vi "Calibration.vi"(8 "error in (no error)":errorcluster) -> (0 "error out":errorcluster, 2 "Cal Success":bool)   [LabVIEW 2018]
uses:
  Microfontest/Peiker_Stepped Sweep Settings.ctl
  <vilib>/addons/_NISVFA/_Shared subVIs/Controls/svc_DSA Channel Settings.ctl
  <vilib>/addons/_NISVFA/_Shared subVIs/Controls/svc_Channel Info.ctl
  <vilib>/addons/_NISVFA/_Shared subVIs/Controls/svc_Engineering Units Text Ring.ctl
  <vilib>/addons/_NISVFA/_Shared subVIs/Controls/svc_Weighting Filter Text Ring.ctl
panel:
  out "FrequencyList Output Level":T1(graph)
  in  "Cancel":bool
  out "calibrated sensor sensitivity [mV/Pa] 2":dbl
  in  "Ret":bool
  in  "Cal":bool
  out "Fundamental Amplitude":T2(graph) caption="Fundamental-Amplitude"
  in  "Freq List file":path=path "D:/Valeo/Micriphone Test/Config/ME79_FreqList_New.csv"
  out "correctedFreqList":T1(array[cluster])
  in  "CalSettings":T3={"SollPegel[dBSPL]"=114, "maxDeviationRef[dB]"=2.0, "maxDeviation[dB]"=2.0, "maxRuns"=20, "RefFrequency[Hz]"=94, "Wait[ms]"=0} {"maxDeviation[dB]" format="%.2f"; "maxDeviationRef[dB]" format="%.2f"}
  out "calibrated sensor sensitivity [mV/Pa]":dbl=nan format="%.2g"
  out "power spectrum":cluster{"x0":dbl, "dx":dbl, "magnitude":dbl[]}(graph)
  in  "calibration settings":T4={"calibration value [dB SPL]"=94.0, "calibration frequency [Hz]"=1000.0}
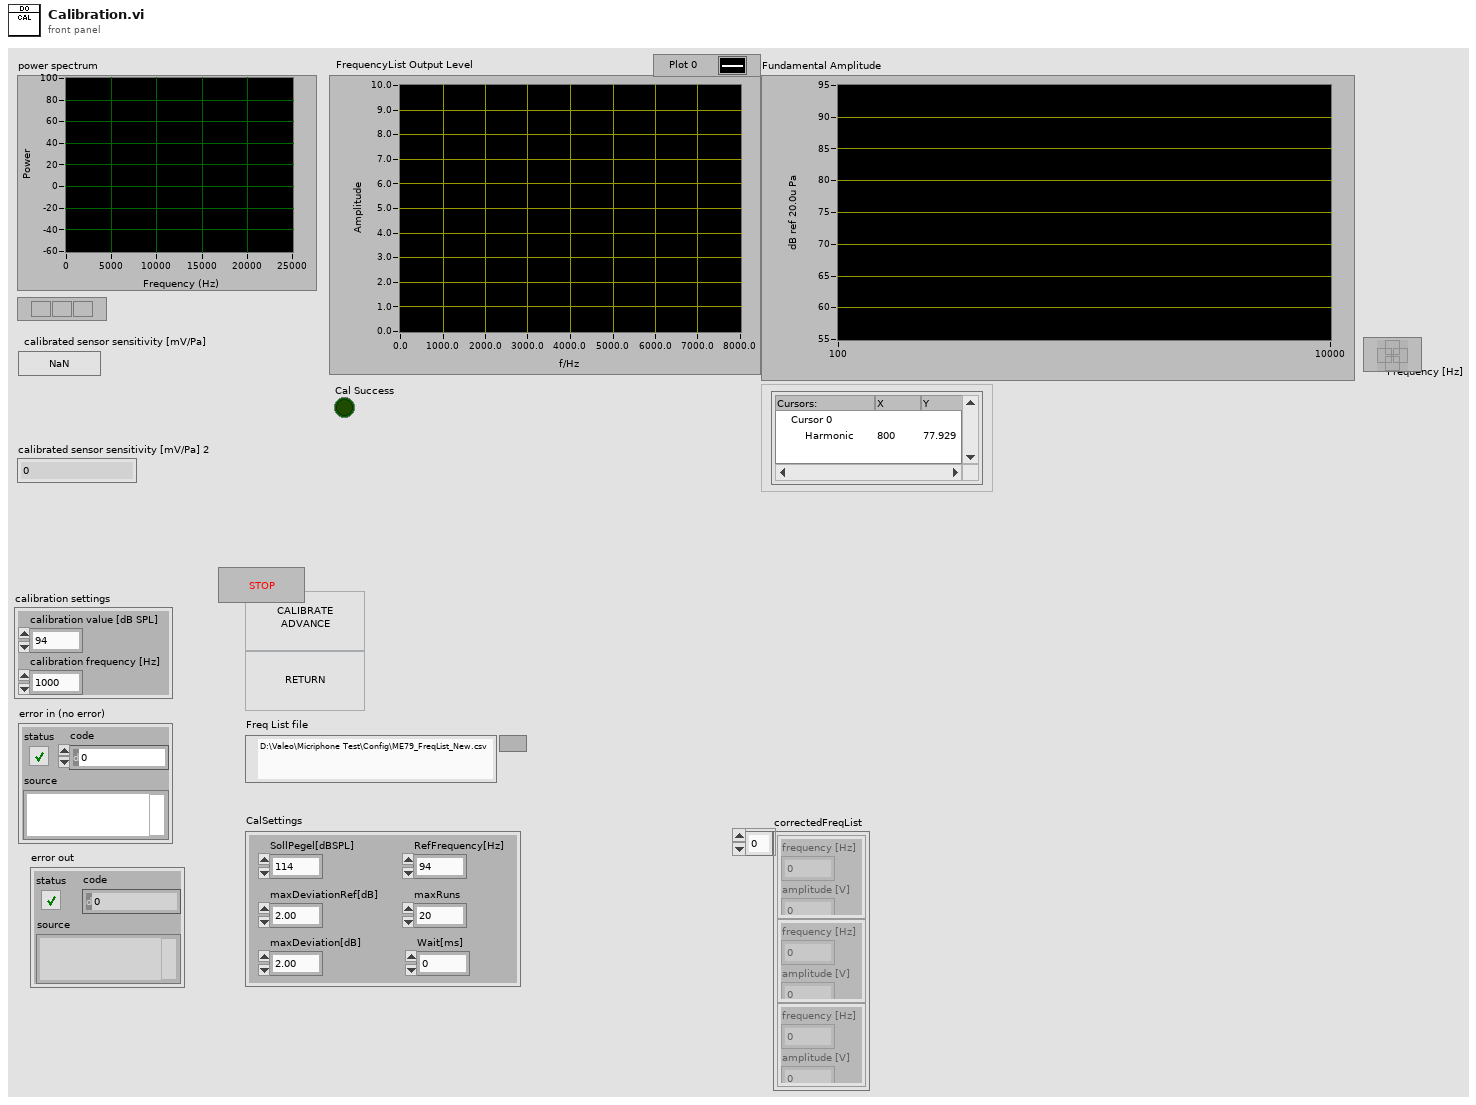
[diagram p1: front panel]
types:
  T1 = cluster{"frequency [Hz]":dbl, "amplitude [V]":dbl}[]
  T2 = cluster{"frequency [Hz]":dbl[], "amplitude":dbl[]}
  T3 = cluster{"SollPegel[dBSPL]":i32, "maxDeviationRef[dB]":dbl, "maxDeviation[dB]":dbl, "maxRuns":i32, "RefFrequency[Hz]":i32, "Wait[ms]":i32}
  T4 = cluster{"calibration value [dB SPL]":dbl, "calibration frequency [Hz]":dbl}
  T5 = typedef "Peiker_Stepped Sweep Settings.ctl" = cluster{"Input Settings":cluster{"IEPE min time to settle [s]":dbl, "Responce Channel Settings":cluster{"DSA response channel settings":T6, "response channel info":T7, "AI response settings":cluster{"response channel":tag, "max value [V]":dbl, "min value [V]":dbl, "terminal configuration":i32}}, "Stimulus Channel Settings":cluster{"AI stimulus settings":cluster{"stimulus channel":tag, "max value [V]":dbl, "min value [V]":dbl, "terminal configuration":i32}, "DSA stimulus channel settings":T6, "stimulus channel info":T7}}, "Output Settings":cluster{"AO source settings":cluster{"excitation channel":tag, "max value [V]":dbl, "min value [V]":dbl, "terminal configuration":i32}}}
  T6 = typedef "svc_DSA Channel Settings.ctl" = cluster{"coupling":i32, "enable IEPE excitation":bool, "IEPE current [mA]":dbl}
  T7 = typedef "svc_Channel Info.ctl" = cluster{"sensor sensitivity":dbl, "engineering units":T8, "dB reference":dbl, "custom label":string, "weighting filter":T9, "pregain":dbl}
  T8 = typedef "svc_Engineering Units Text Ring.ctl" = u16
  T9 = typedef "svc_Weighting Filter Text Ring.ctl" = u16
  T10 = enum16{"Left Button", "Center Button", "Right Button", "Window Close"}
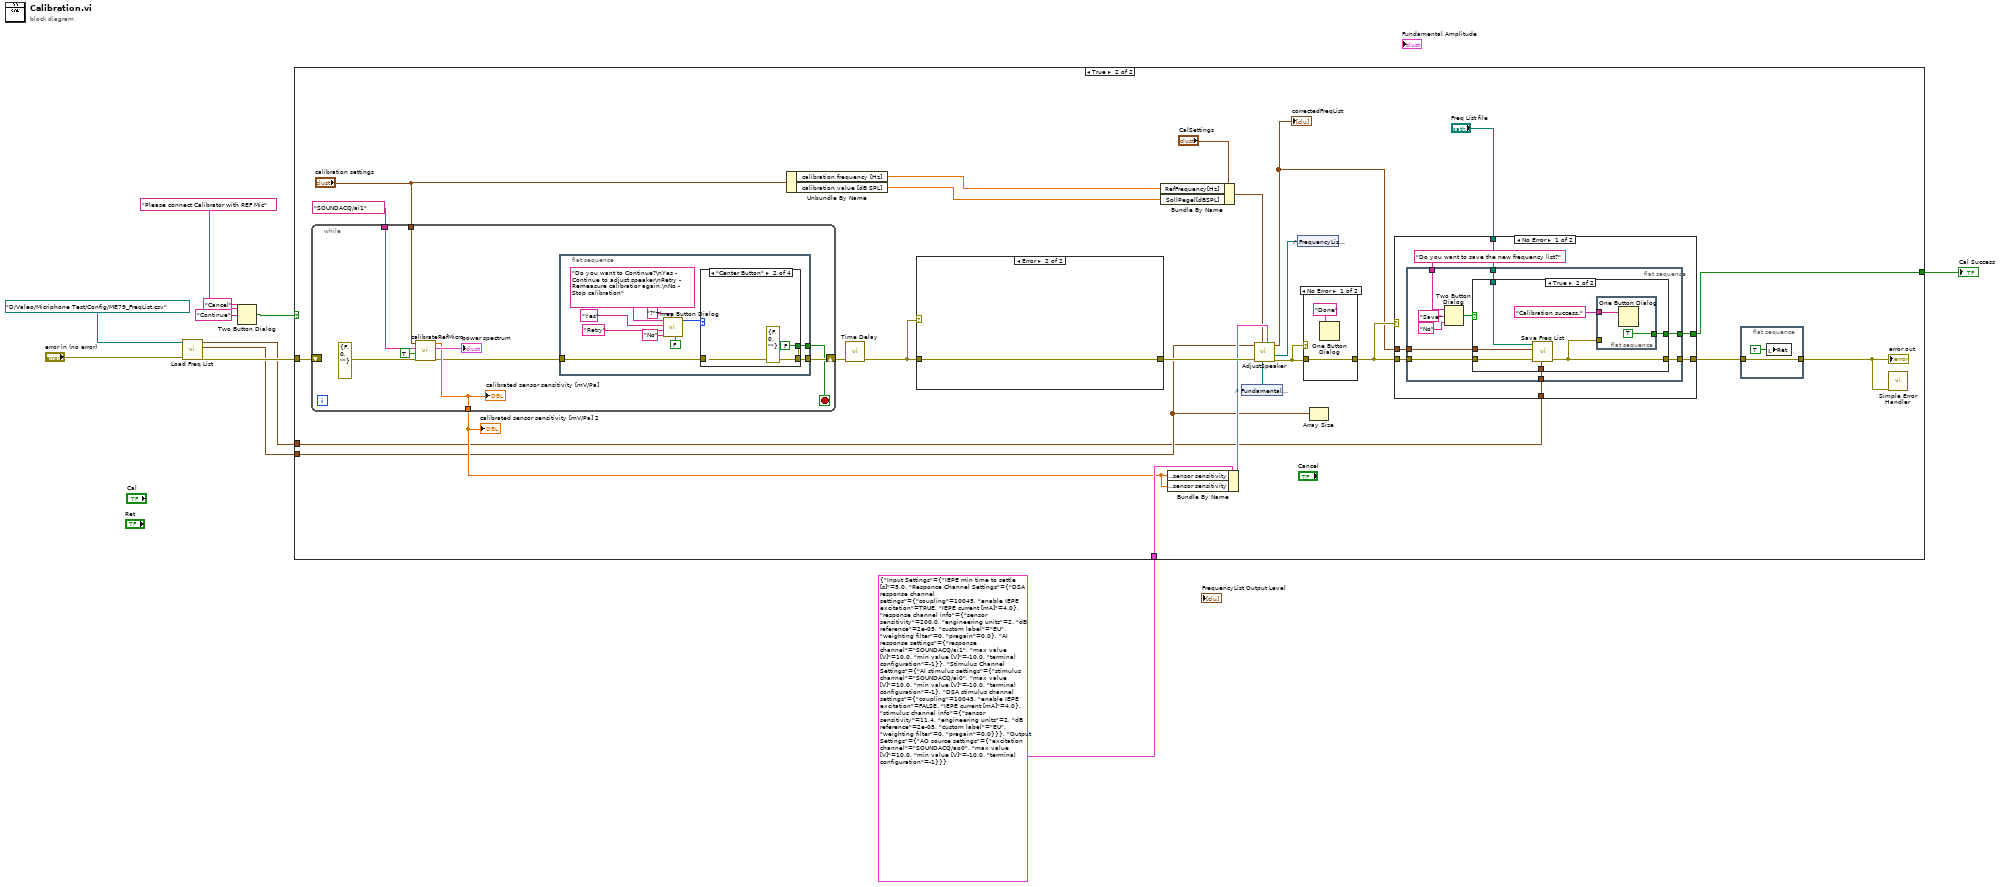
[diagram p0: block diagram]
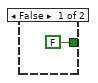
[diagram p2: hidden frame]
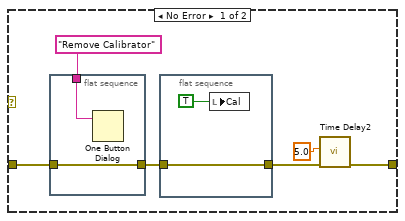
[diagram p3: hidden frame]
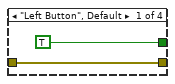
[diagram p4: hidden frame]
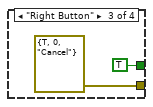
[diagram p5: hidden frame]
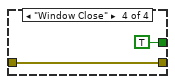
[diagram p6: hidden frame]
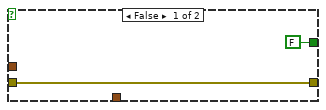
[diagram p7: hidden frame]
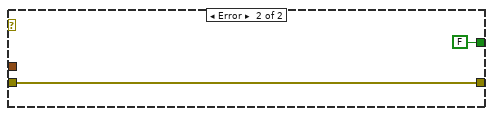
[diagram p8: hidden frame]
diagram:
  n1 = call "Load Freq List.vi"("error in (no error)"="error in (no error)", "Freq List file"=path "D:/Valeo/Micriphone Test/Config/ME79_FreqList.csv" ("dup path")) -> ("error out"=w7:errorcluster, "Frequency List"=w6:T1, "Spec List"=w1:cluster{"Lower":dbl, "Upper":dbl}[])  [unwired: 5 in, 2 out]
  n2 = Two Button Dialog(message="Please connect Calibrator with REF Mic", 1:"Cancel" ("F button name (\"Cancel\")"), 2:"Continue" ("T button name (\"OK\")")) -> (T button?=w10:bool)
  n3 = case shown="True" w10 {
    tunnel: w7 -> [_ w31]
    tunnel: w6 -> [_ w15]
    tunnel: T5 {"Input Settings"={"IEPE min time to settle [s]"=5.0, "Responce Channel Settings"={"DSA response channel settings"={"coupling"=10045, "enable IEPE excitation"=TRUE, "IEPE current [mA]"=4.0}, "response channel info"={"sensor sensitivity"=200.0, "engineering units"=2, "dB reference"=2e-05, "custom label"="EU", "weighting filter"=0, "pregain"=0.0}, "AI response settings"={"response channel"="SOUNDACQ/ai1", "max value [V]"=10.0, "min value [V]"=-10.0, "terminal configuration"=-1}}, "Stimulus Channel Settings"={"AI stimulus settings"={"stimulus channel"="SOUNDACQ/ai0", "max value [V]"=10.0, "min value [V]"=-10.0, "terminal configuration"=-1}, "DSA stimulus channel settings"={"coupling"=10045, "enable IEPE excitation"=FALSE, "IEPE current [mA]"=4.0}, "stimulus channel info"={"sensor sensitivity"=11.4, "engineering units"=2, "dB reference"=2e-05, "custom label"="EU", "weighting filter"=0, "pregain"=0.0}}}, "Output Settings"={"AO source settings"={"excitation channel"="SOUNDACQ/ao0", "max value [V]"=10.0, "min value [V]"=-10.0, "terminal configuration"=-1}}} ("Peiker_Stepped Sweep Settings") -> [_ w33]
    tunnel: [FALSE w17] -> w4
    tunnel: w1 -> [_ w14]
    frame False {
    }
    frame True {
      n4 = while {
        tunnel: tag "SOUNDACQ/ai1" ("DAQmx physical channel") -> [w56]
        tunnel: [w53] -> w30
        tunnel: "calibration settings" -> [w52]
        shift-right: [w49] -> w35
        shift-left: w31 -> [_]
        stop <- w50 stop-if-true
        n5 = call "calibrateRefMicro.vi"("error in (no error)"=errorcluster {"status"=FALSE, "code"=0, "source"=""} ("error out"), "enable IEPE excitation (F)"=TRUE, "DAQmx physical channel"=w56, "calibration settings"=w52) -> ("error out"=w51:errorcluster, "power spectrum"=→"power spectrum":cluster{"x0":dbl, "dx":dbl, "magnitude":dbl[]}, "calibrated sensor sensitivity [mV/Pa]"=w53:dbl)  [unwired: 5 in]
        "calibrated sensor sensitivity [mV/Pa]" <- w53
        n6 = flat-sequence {
          tunnel: w51 -> [w58]
          tunnel: [w59] -> w50
          tunnel: [w57] -> w49
          frame #0 {
            n7 = call <vilib>:"Three Button Dialog.vi"("Allow user to close window? (TRUE)"=FALSE, "Window Title (\"\")"="?" ("Window Title (\"\")"), "Right Button Text (\"Cancel\")"="No" ("Right Button Text (\"Cancel\")"), "Center Button Text (\"No\")"="Retry" ("Center Button Text (\"No\")"), "Left Button Text (\"Yes\")"="Yes" ("Left Button Text (\"Yes\")"), "message"="Do you want to Continue?\nYes - Continue to adjust speaker\nRetry - Remeasure calibratior again.\nNo - Stop calibration") -> ("Which Button?"=w60:T10)  [unwired: 5 in]
            n8 = case shown="\"Center Button\"" w60 {
              tunnel: [TRUE FALSE TRUE TRUE] -> w59
              tunnel: w58 -> [w67 _ _ w74]
              tunnel: [w67 errorcluster {"status"=FALSE, "code"=0, "source"=""} ("error out") errorcluster {"status"=TRUE, "code"=0, "source"="Cancel"} ("error out") w74] -> w57
              frame "Left Button", Default {
              }
              frame "Center Button" {
              }
              frame "Right Button" {
              }
              frame "Window Close" {
              }
            }
          }
        }
      }
      "calibrated sensor sensitivity [mV/Pa] 2" <- w30
      n9 = Unbundle By Name("calibration settings") -> ("calibration frequency [Hz]"=w26:dbl, "calibration value [dB SPL]"=w25:dbl)
      n10 = call "Time Delay"("error in (no error)"=w35) -> ("error out"=w18:errorcluster)  [unwired: 10 in]
      n11 = case shown="Error" w18 {
        tunnel: w18 -> [w42 w47]
        tunnel: [w40 w47] -> w34
        frame No Error {
          n12 = flat-sequence {
            tunnel: w42 -> [w46]
            tunnel: [w46] -> w38
            tunnel: "Remove Calibrator" -> [w45]
            frame #0 {
              n13 = One Button Dialog(message=w45) -> ()  [unwired: 1 in, 1 out]
            }
          }
          n14 = flat-sequence {
            tunnel: w38 -> [w43]
            tunnel: [w43] -> w37
            frame #0 {
              n15 = local write "Cal"(TRUE ("Adv 3")) -> ()
            }
          }
          n16 = call "Time Delay2"("error in (no error)"=w37, "Delay Time (s)"=5.0) -> ("error out"=w40:errorcluster)  [unwired: 9 in]
        }
        frame Error {
        }
      }
      n17 = Bundle By Name(cluster="CalSettings", "RefFrequency[Hz]"=w26, "SollPegel[dBSPL]"=w25) -> (w24:T3)
      n18 = Bundle By Name(cluster=w33, "Input Settings.Responce Channel Settings.response channel info.sensor sensitivity"=w30, "Input Settings.Stimulus Channel Settings.stimulus channel info.sensor sensitivity"=w30) -> (w32:T5)
      n19 = control-ref of="Fundamental Amplitude"() -> (w29:refnum<vi>)
      n20 = control-ref of="FrequencyList Output Level"() -> (w13:refnum<vi>)
      n21 = call "AdjustSpeaker.vi"("Input Signal"=w13, "Peiker_Stepped Sweep Settings"=w32, "Fundamental Amplitude 2"=w29, "CalSettings"=w24, "error in"=w34, "Frequency List"=w15) -> ("error out"=w23:errorcluster, "correctedFreqList"=w20:T1)  [unwired: 3 in, 1 out]
      "correctedFreqList" <- w20
      n22 = case shown="No Error" w23 {
        tunnel: w23 -> [w107 w109]
        tunnel: [w107 w109] -> w22
        frame No Error {
          n23 = One Button Dialog(message="Done") -> ()  [unwired: 1 in, 1 out]
        }
        frame Error {
        }
      }
      n24 = Array Size(array=w15) -> ()  [unwired: 1 out]
      n25 = case shown="No Error" w22 {
        tunnel: w22 -> [w83 w106]
        tunnel: [w81 w106] -> w19
        tunnel: "Freq List file" -> [w80 _]
        tunnel: w20 -> [w79 _]
        tunnel: [w78 FALSE] -> w17
        tunnel: w14 -> [w77 _]
        frame No Error {
          n26 = flat-sequence {
            tunnel: w83 -> [w90]
            tunnel: "Do you want to save the new frequency list?" -> [w93]
            tunnel: [w88] -> w81
            tunnel: w80 -> [w87]
            tunnel: w79 -> [w86]
            tunnel: [w85] -> w78
            tunnel: w77 -> [w84]
            frame #0 {
              n27 = Two Button Dialog(message=w93, 1:"No" ("T button name (\"OK\")"), 2:"Save" ("T button name (\"OK\")")) -> (T button?=w89:bool)
              n28 = case shown="True" w89 {
                tunnel: w90 -> [w95 w102]
                tunnel: [w95 w99] -> w88
                tunnel: w87 -> [_ w101]
                tunnel: w86 -> [_ w100]
                tunnel: [FALSE w97] -> w85
                tunnel: w84 -> [_ w96]
                frame False {
                }
                frame True {
                  n29 = call "Save Freq List.vi"("Spec List"=w96, "error in (no error)"=w102, "correctedFreqList"=w100, "Freq List file"=w101) -> ("error out"=w99:errorcluster)  [unwired: 7 in]
                  n30 = flat-sequence {
                    tunnel: w99 -> [_]
                    tunnel: "Calibration success." -> [w104]
                    tunnel: [TRUE] -> w97
                    frame #0 {
                      n31 = One Button Dialog(message=w104) -> ()  [unwired: 1 in, 1 out]
                    }
                  }
                }
              }
            }
          }
        }
        frame Error {
        }
      }
      n32 = flat-sequence {
        tunnel: w19 -> [w75]
        tunnel: [w75] -> w16
        frame #0 {
          n33 = local write "Ret"(TRUE ("Adv 2")) -> ()
        }
      }
      n34 = call <vilib>:"Simple Error Handler.vi"("error in (no error)"=w16) -> ()  [unwired: 4 in, 5 out]
      "error out" <- w16
    }
  }
  "Cal Success" <- w4
